vi "未命名 3.vi"() -> ()   [LabVIEW 2020]
panel:
  in  "文本下拉列表":u16(ring)
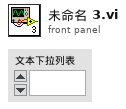
[diagram p1: front panel]
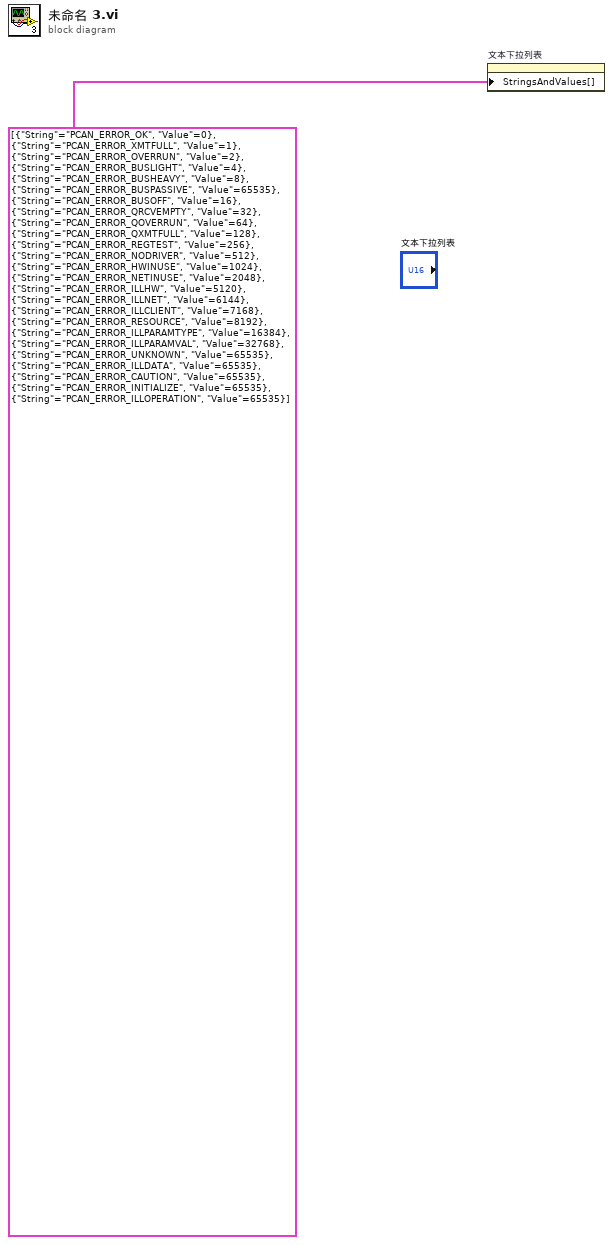
[diagram p0: block diagram]
diagram:
  n1 = property on="文本下拉列表" class="Ring (严格)"("StringsAndValues[]"=cluster{"String":string, "Value":u16}[] [{"String"="PCAN_ERROR_OK", "Value"=0}, {"String"="PCAN_ERROR_XMTFULL", "Value"=1}, {"String"="PCAN_ERROR_OVERRUN", "Value"=2}, {"String"="PCAN_ERROR_BUSLIGHT", "Value"=4}, {"String"="PCAN_ERROR_BUSHEAVY", "Value"=8}, {"String"="PCAN_ERROR_BUSPASSIVE", "Value"=65535}, {"String"="PCAN_ERROR_BUSOFF", "Value"=16}, {"String"="PCAN_ERROR_QRCVEMPTY", "Value"=32}, {"String"="PCAN_ERROR_QOVERRUN", "Value"=64}, {"String"="PCAN_ERROR_QXMTFULL", "Value"=128}, {"String"="PCAN_ERROR_REGTEST", "Value"=256}, {"String"="PCAN_ERROR_NODRIVER", "Value"=512}, {"String"="PCAN_ERROR_HWINUSE", "Value"=1024}, {"String"="PCAN_ERROR_NETINUSE", "Value"=2048}, {"String"="PCAN_ERROR_ILLHW", "Value"=5120}, {"String"="PCAN_ERROR_ILLNET", "Value"=6144}, {"String"="PCAN_ERROR_ILLCLIENT", "Value"=7168}, {"String"="PCAN_ERROR_RESOURCE", "Value"=8192}, {"String"="PCAN_ERROR_ILLPARAMTYPE", "Value"=16384}, {"String"="PCAN_ERROR_ILLPARAMVAL", "Value"=32768}, {"String"="PCAN_ERROR_UNKNOWN", "Value"=65535}, {"String"="PCAN_ERROR_ILLDATA", "Value"=65535}, {"String"="PCAN_ERROR_CAUTION", "Value"=65535}, {"String"="PCAN_ERROR_INITIALIZE", "Value"=65535}, {"String"="PCAN_ERROR_ILLOPERATION", "Value"=65535}] ("数组")) -> ()  [unwired: 2 in, 2 out]
